vi "Read Left Child Node.vi"(8 "error in (no error)":errorcluster, 11 "Formula Phrasing Binary Tree Node in":refnum<class "Formula Phrasing Binary Tree Node.lvclass">) -> (0 "error out":errorcluster, 2 "Math Formula String Phrasing.lvclass":refnum<class "Math Formula String Phrasing.lvclass">, 3 "Formula Phrasing Binary Tree Node out":refnum<class "Formula Phrasing Binary Tree Node.lvclass">)   [LabVIEW 2024, in "Formula Phrasing Binary Tree Node.lvclass"]
uses:
  Formula Phrasing Binary Tree Node.lvclass
  Math Formula String Phrasing/Math Formula String Phrasing.lvclass
  Formula Phrasing Binary Tree Node.lvclass/Formula Phrasing Binary Tree Node.ctl
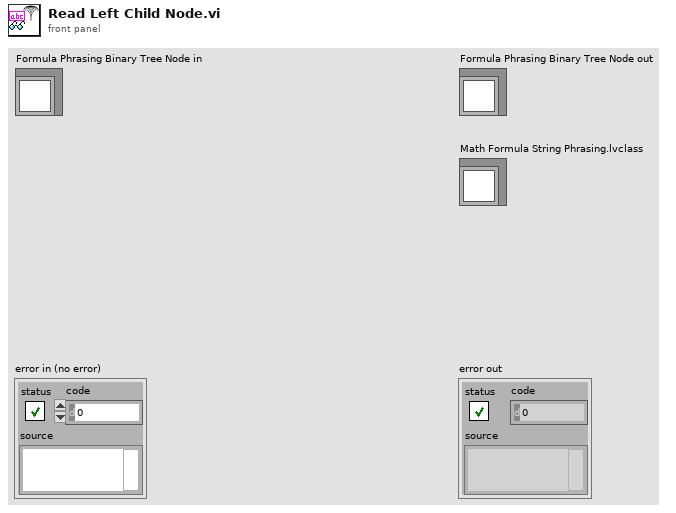
[diagram p1: front panel]
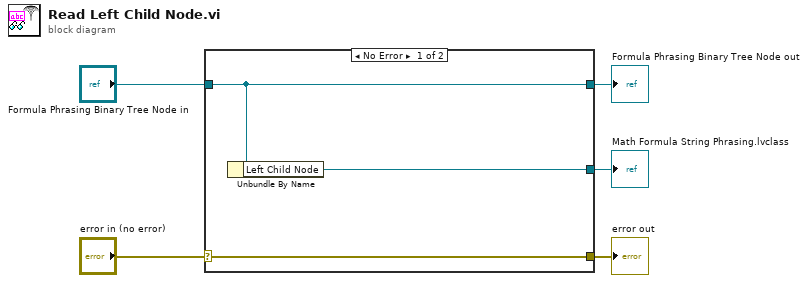
[diagram p0: block diagram]
diagram:
  n1 = case shown="No Error" "error in (no error)" {
    selector: "error in (no error)" -> [w8 w9]
    tunnel: [w8 w9] -> w4
    tunnel: [w7 w10] -> w2
    tunnel: "Formula Phrasing Binary Tree Node in" -> [w7 w10]
    tunnel: [w6 _] -> w1
    frame No Error {
      n2 = Unbundle By Name(w7) -> ("Left Child Node"=w6:refnum<class "Math Formula String Phrasing.lvclass">)
    }
    frame Error {
    }
  }
  "error out" <- w4
  "Formula Phrasing Binary Tree Node out" <- w2
  "Math Formula String Phrasing.lvclass" <- w1
